vi "CCE T027 SubVI03.vi"(9 "q":dbl, 10 "p":dbl, 11 "Image Data":u8[][](array[numeric])) -> (3 "M. Inicial":dbl)   [LabVIEW 2020]
doc: "Ceballos Conde Emanuel 4MV6 Sistemas de visión artificial 2022/1\neste vi permite obtener el momento inicial de una imagen previamente binarizada"
panel:
  # "Ceballos Conde Emanuel\n4MV6\nSistemas de visión artificial\n2022/1"
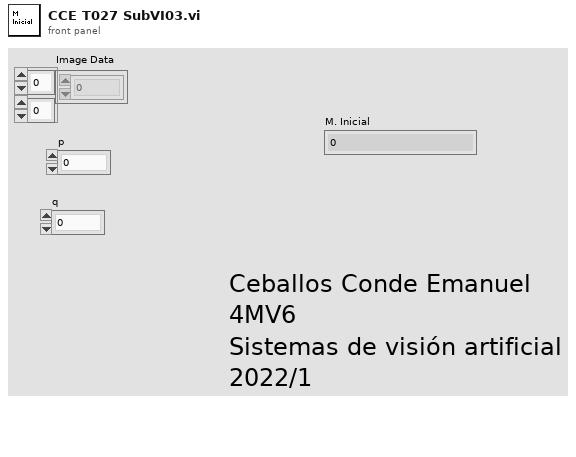
[diagram p1: front panel]
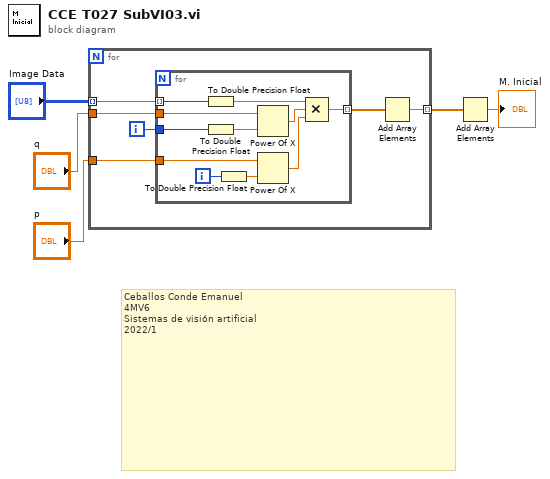
[diagram p0: block diagram]
diagram:
  # "Ceballos Conde Emanuel\n4MV6\nSistemas de visión artificial\n2022/1"
  n1 = for {
    tunnel: "Image Data" -> [w11] mode=indexing
    tunnel: "q" -> [w10]
    tunnel: "p" -> [w9]
    tunnel: [w6] -> w4 mode=indexing
    i -> [w8]
    n2 = for {
      tunnel: w11 -> [w18] mode=indexing
      tunnel: w10 -> [w22]
      tunnel: w9 -> [w21]
      tunnel: w8 -> [w14]
      tunnel: [w12] -> w7 mode=indexing
      i -> [w16]
      n3 = To Double Precision Float(number=w18) -> (double precision float=w13:dbl)
      n4 = To Double Precision Float(number=w14) -> (double precision float=w15:dbl)
      n5 = To Double Precision Float(number=w16) -> (double precision float=w17:dbl)
      n6 = Power Of X(1:w15, 2:w22) -> (0:w20:dbl)
      n7 = Power Of X(1:w17, 2:w21) -> (0:w19:dbl)
      n8 = Compound Arithmetic op=MULTIPLY(w13, w20, w19) -> (w12:dbl)
    }
    n9 = Add Array Elements(numeric array=w7) -> (sum=w6:dbl)
  }
  n10 = Add Array Elements(numeric array=w4) -> (sum=→"M. Inicial":dbl)
